vi "Import Table.vi"(8 "error in (no error)":errorcluster, 10 "Tables":string, 11 "MYSQL Database in":refnum<class "MYSQL Database.lvclass">) -> (0 "error out":errorcluster, 3 "MYSQL Database out":refnum<class "MYSQL Database.lvclass">)   [LabVIEW 2023, in "HardwareAbstractionLayer_LVOOP.lvlib" / "MYSQL Database.lvclass"]
uses:
  MYSQL Database.lvclass
  SQL Public VI/Control/DB Options.ctl
  <vilib>/Utility/file.llb/Read Delimited Spreadsheet (string).vi
  Database.lvclass
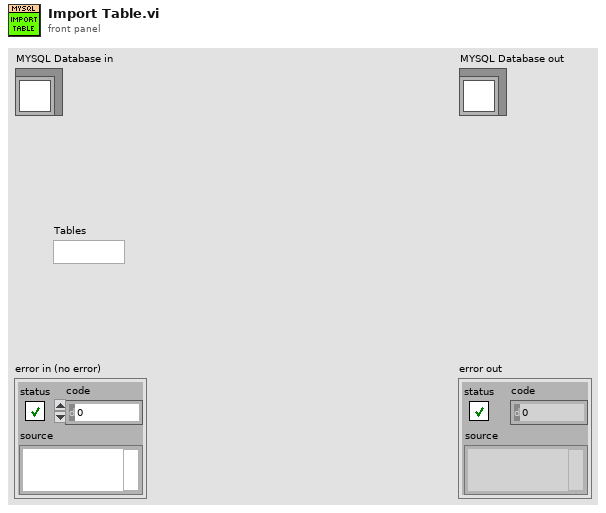
[diagram p1: front panel]
types:
  T1 = cluster{"table":string, "columns":string[], "Data":string[][], "Schema Name":string}
  T2 = typedef "HardwareAbstractionLayer_LVOOP.lvlib/Database.lvclass/DB Options.ctl" = enum16{"Init", "Select Data", "Insert Data", "Update Data", "Delete Data", "Execute Query", "Create Schema", "Create Table", "List Tables", "List Columns", "Close"}
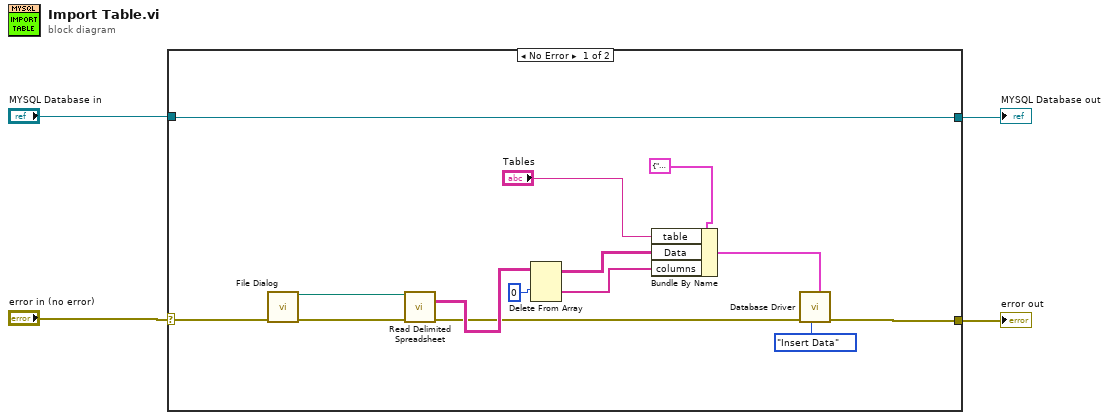
[diagram p0: block diagram]
diagram:
  n1 = case shown="No Error" "error in (no error)" {
    selector: "error in (no error)" -> [w8 w20]
    tunnel: [w7 w20] -> w3
    tunnel: "MYSQL Database in" -> [w9 w19]
    tunnel: [w9 w19] -> w1
    frame No Error {
      n2 = call "File Dialog"("error in"=w8) -> ("selected path"=w11:path, "error out"=w12:errorcluster)  [unwired: 11 in, 2 out]
      n3 = call-poly <vilib>:"Read Delimited Spreadsheet.vi"("file path (dialog if empty)"=w11, "error in (no error)"=w12) -> ("all rows"=w17:string[][], "error out"=w13:errorcluster)  [unwired: 8 in, 4 out]
      n4 = Delete From Array(array=w17, index (row)=0) -> (deleted portion=w15:string[], array with subset deleted=w16:string[][])  [unwired: 2 in]
      n5 = Bundle By Name(cluster=T1 {"table"="", "columns"=[], "Data"=[], "Schema Name"=""} ("Insert Data"), "table"="Tables", "Data"=w16, "columns"=w15) -> (w5:T1)
      n6 = call "Database Driver.vi"("Insert Data"=w5, "Options"=DB_Options."Insert Data", "error in"=w13) -> ("error out"=w7:errorcluster)  [unwired: 5 in, 3 out]
    }
    frame Error {
    }
  }
  "error out" <- w3
  "MYSQL Database out" <- w1
